vi "Session Read.vi"(8 "error in (no error)":errorcluster, 10 "Timeout":i32=5000, 11 "HSMS Class in":refnum<class "HSMS Class.lvclass">) -> (0 "error out":errorcluster, 2 "Message Packet":T1, 3 "HSMS Class out":refnum<class "HSMS Class.lvclass">)   [LabVIEW 2020, in "SECS Communication.lvlib" / "HSMS Class.lvclass"]
uses:
  HSMS Class.lvclass
  Message Packet.ctl
  HSMS Class.lvclass/HSMS Class.ctl
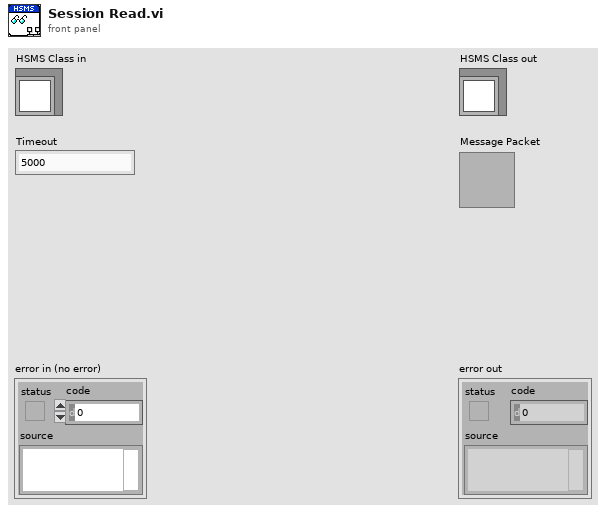
[diagram p1: front panel]
types:
  T1 = typedef "SECS Communication.lvlib/HSMS Class.lvclass/Message Packet.ctl" = cluster{"Message Header Cluster":T2, "Message Header":u8[], "Message Text":u8[]}
  T2 = typedef "SECS Communication.lvlib/HSMS Class.lvclass/Message Header.ctl" = cluster{"Byte 0-1(Session ID)":u16, "W-Bit":bool, "Byte 2":u8, "Byte 3":u8, "Byte 4(PType)":T3, "Byte 5(SType)":T4, "Byte 6-9(System Btyes)":u8[]}
  T3 = typedef "SECS Communication.lvlib/HSMS Class.lvclass/PType.ctl" = enum8{"SECS-II Encoding", "Reserved"}
  T4 = typedef "SECS Communication.lvlib/HSMS Class.lvclass/SType.ctl" = enum8{"Data Message", "Select.req", "Select.rsp", "Deselect.req", "Deselect.rsp", "Linktest.req", "Linktest.rsp", "Reject.req", "Separate.req"}
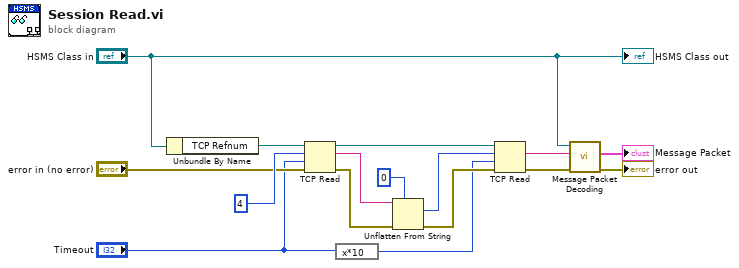
[diagram p0: block diagram]
diagram:
  n1 = Unbundle By Name("HSMS Class in") -> ("TCP Refnum"=w9:refnum<k5>)
  n2 = TCP Read(connection ID=w9, bytes to read=4, error in (no error)="error in (no error)", 9:"Timeout") -> (connection ID out=w13:refnum<k5>, data out=w8:string, error out=w14:errorcluster)  [unwired: 1 out]
  n3 = expression code="x*10"("Timeout") -> (w1:i32)
  n4 = Unflatten From String(type=0 ("bytes to read"), binary string=w8, error in (no error)=w14) -> (value=w12:i32, error out=w11:errorcluster)  [unwired: 1 in, 2 out]
  n5 = TCP Read(connection ID=w13, bytes to read=w12, error in (no error)=w11, 9:w1) -> (data out=w6:string, error out=w7:errorcluster)  [unwired: 2 out]
  n6 = call "Message Packet Decoding.vi"("error in (no error)"=w7, "Data"=w6, "HSMS Class in"="HSMS Class in") -> ("error out"=→"error out":errorcluster, "Message Packet"=→"Message Packet":T1)  [unwired: 6 in, 1 out]
  "HSMS Class out" <- "HSMS Class in"
